vi "Process single turn magnet data.vi"(6 "Save data":bool=TRUE, 7 "Offset correction":dbl, 8 "Error In":errorcluster, 9 "Offset duration":dbl=1e-06, 10 "Integration settings":T1={"Channel"="", "Output name"="", "Factor"=1.0, "Start time"=0.0, "Duration"=0.0, "Fix drift"=FALSE} {"Duration" format="%#_6ps"; "Start time" format="%#_6ps"}, 11 "File Path Control":path) -> (0 "Error Out":errorcluster, 2 "Min max":cluster{"Max":dbl, "Min":dbl}, 3 "Waveform Graph":waveform(dbl)(graph))   [LabVIEW 2016]
uses:
  Libraries/Utilities/Controls/Integrate channel.ctl
panel:
  # "Bdot name"
  # "Factor"
  # "Output name"
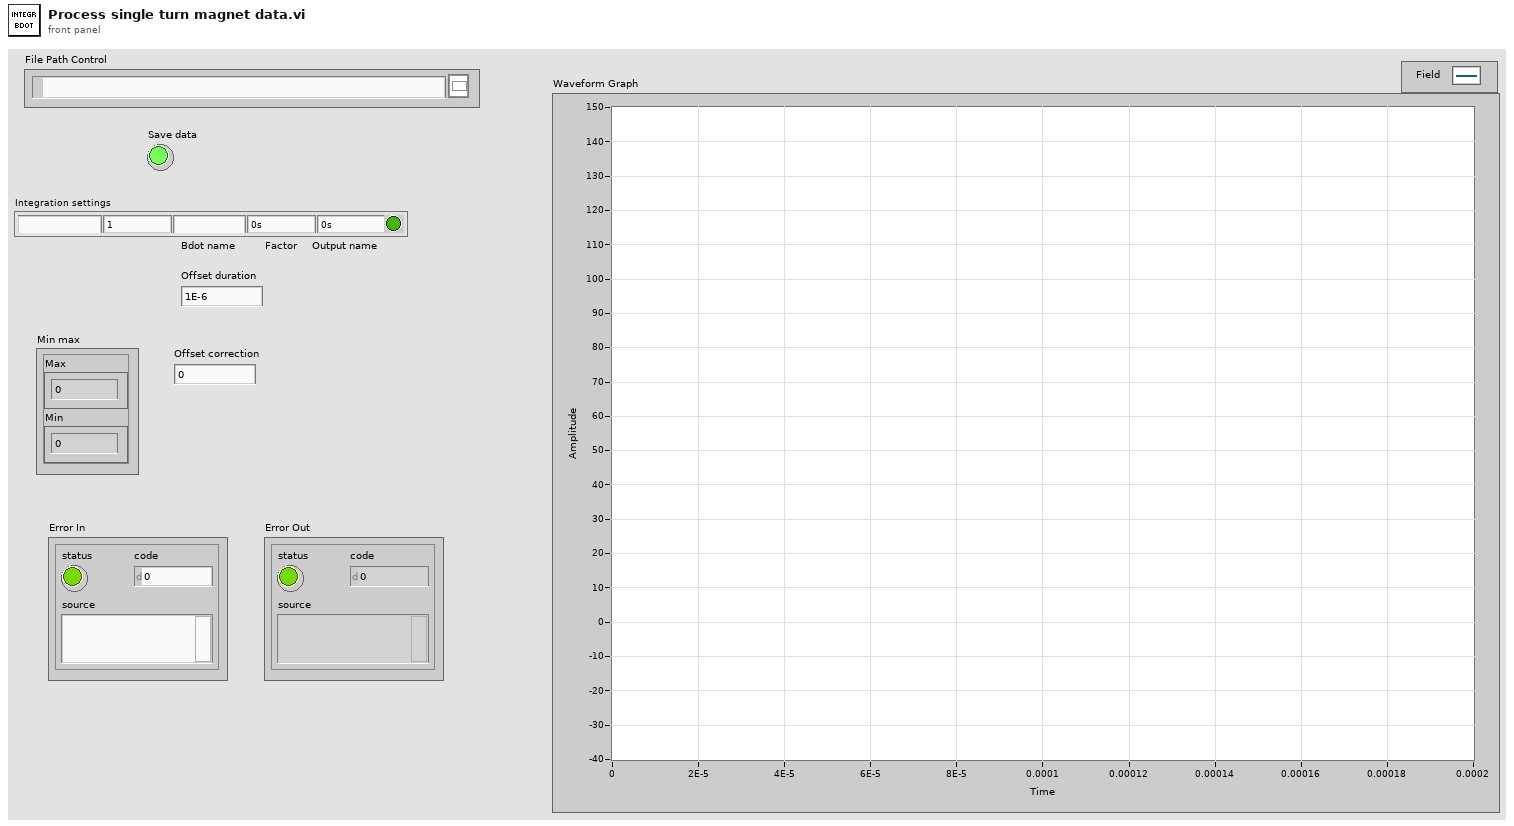
[diagram p1: front panel]
types:
  T1 = typedef "Integrate channel.ctl" = cluster{"Channel":string, "Output name":string, "Factor":dbl, "Start time":dbl, "Duration":dbl, "Fix drift":bool}
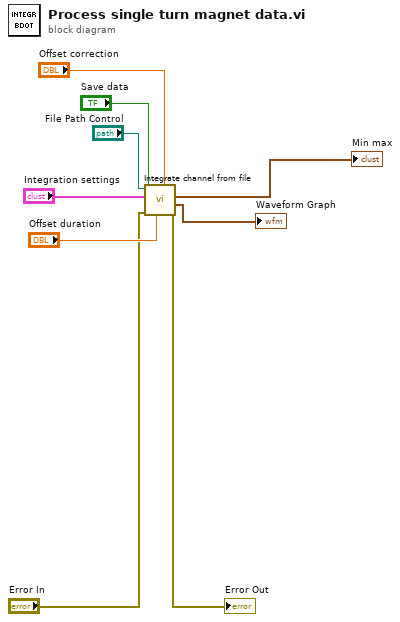
[diagram p0: block diagram]
diagram:
  n1 = call "Integrate channel from file.vi"("Offset correction"="Offset correction", "Offset duration"="Offset duration", "Error In"="Error In", "Save data"="Save data", "Integration settings"="Integration settings", "File Path Control"="File Path Control") -> ("Error Out"=→"Error Out":errorcluster, "Integrated Waveform"=→"Waveform Graph":waveform(dbl), "Min max"=→"Min max":cluster{"Max":dbl, "Min":dbl})  [unwired: 2 in, 1 out]
